vi "AutoIndent.vi"(7 "Python Code":refnum<vi>, 11 "NewVal in":string) -> (3 "NewVal out":string)   [LabVIEW 2020]
uses:
  <vilib>/Utility/miscctls.llb/LVSelectionTypeDef.ctl
panel:
  out "prev line":string
  out "Text.Selection":T1
  out "indent":i32
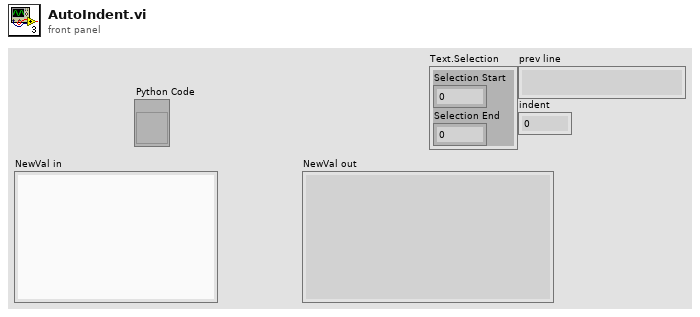
[diagram p1: front panel]
types:
  T1 = typedef "LVSelectionTypeDef.ctl" = cluster{"Selection Start":u32, "Selection End":u32}
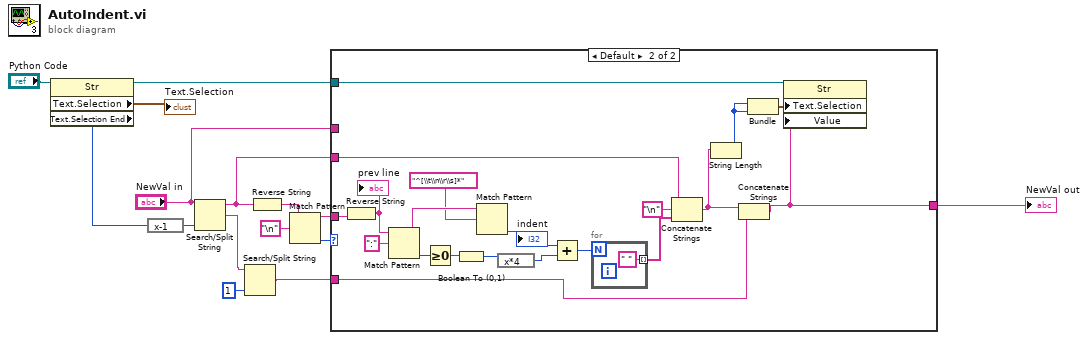
[diagram p0: block diagram]
diagram:
  n1 = property class="Str"(reference="Python Code") -> (reference out=w1:refnum<vi>, "Text.Selection"=→"Text.Selection":T1, "Text.Selection End"=w8:u32)  [unwired: 1 in, 1 out]
  n2 = expression code="x-1"(w8) -> (w7:u32)
  n3 = Search/Split String(string="NewVal in", offset (0)=w7) -> (substring before match=w6:string, match + rest of string=w5:string)  [unwired: 1 in, 1 out]
  n4 = Search/Split String(string=w5, offset (0)=1) -> (match + rest of string=w3:string)  [unwired: 1 in, 2 out]
  n5 = Reverse String(1:w6) -> (0:w11:string)
  n6 = Match Pattern(string=w11, regular expression="\n") -> (before substring=w10:string, offset past match=w9:i32)  [unwired: 1 in, 2 out]
  n7 = case shown="Default" w9 {
    tunnel: w10 -> [_ w36]
    tunnel: [w16 w17] -> w14
    tunnel: w6 -> [_ w24]
    tunnel: w3 -> [_ w20]
    tunnel: "NewVal in" -> [w16 _]
    tunnel: w1 -> [_ w22]
    frame 0 {
    }
    frame Default {
      n8 = Reverse String(1:w36) -> (0:w35:string)
      "prev line" <- w35
      n9 = Match Pattern(string=w35, regular expression=":") -> (before substring=w32:string, offset past match=w33:i32)  [unwired: 1 in, 2 out]
      n10 = Greater Or Equal To 0?(x=w33) -> (x >= 0?=w30:bool)
      n11 = Boolean To (0,1)(Boolean=w30) -> (0, 1=w29:i16)
      n12 = Match Pattern(string=w32, regular expression="^[\\t\\n\\r\\s]*") -> (offset past match=w27:i32)  [unwired: 1 in, 3 out]
      "indent" <- w27
      n13 = expression code="x*4"(w29) -> (w28:i16)
      n14 = Add(x=w27, y=w28) -> (x+y=w26:i32)
      n15 = for {
        N: w26 -> [_]
        tunnel: [" " ("regular expression")] -> w25 mode=indexing
      }
      n16 = Concatenate Strings(w24, "\n" ("string"), w25) -> (w21:string)
      n17 = String Length(string=w21) -> (length=w19:i32)
      n18 = Concatenate Strings(w21, w20) -> (w17:string)
      n19 = Bundle(w19, w19) -> (w18:cluster{i32, i32})  [unwired: 1 in]
      n20 = property class="Str"(reference=w22, "Text.Selection"=w18, "Value"=w17) -> ()  [unwired: 1 in, 2 out]
    }
  }
  "NewVal out" <- w14
